vi "Run VI Asynchronously.vi"() -> ()   [LabVIEW 2019, in "Architecture.lvlib"]
uses:
  Architecture.lvlib
  Modules/Module Template/Module Template.lvlib
panel:
  out "error out":errorcluster
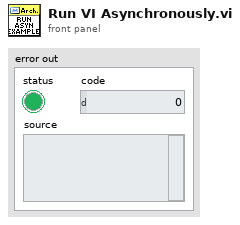
[diagram p1: front panel]
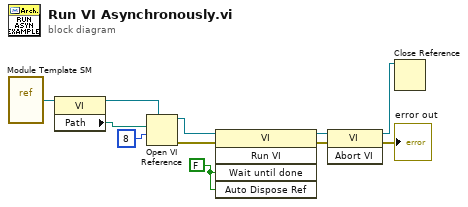
[diagram p0: block diagram]
diagram:
  w8 = FALSE ("Wait Until Done")
  n1 = vi-ref "Module Template SM.vi"() -> (w7:refnum<vi>)
  n2 = property class="VI"(reference=w7) -> (reference out=w6:refnum<vi>, "Path"=w5:path)  [unwired: 1 in, 1 out]
  n3 = Open VI Reference(type specifier VI Refnum (for type only)=w6, vi path=w5, options=8) -> (vi reference=w9:refnum<vi>, error out=w10:errorcluster)  [unwired: 3 in]
  n4 = invoke class="VI" method="Run VI"(reference=w9, error in=w10, "Wait until done"=w8, "Auto Dispose Ref"=w8) -> (reference out=w4:refnum<vi>, error out=w3:errorcluster)  [unwired: 1 in, 3 out]
  n5 = invoke class="VI" method="Abort VI"(reference=w4, error in=w3) -> (reference out=w1:refnum<vi>, error out=→"error out":errorcluster)  [unwired: 1 in, 1 out]
  n6 = Close Reference(reference=w1) -> ()  [unwired: 1 in, 1 out]
